vi "Get Cursor Position.vi"(8 "Logarithm?":bool, 9 "Inverted?":bool, 10 "Range":cluster{"Max":sgl, "Min":sgl}, 11 "Cursor Value In":sgl) -> (3 "Cursor Value Out":sgl)   [LabVIEW 2017, in "3D Plot.lvclass"]
uses:
  <vilib>/Math Plots/3D Math Plots/3D Plot/3D Plot/3D Plot.lvclass
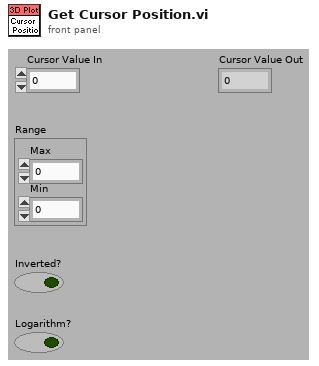
[diagram p1: front panel]
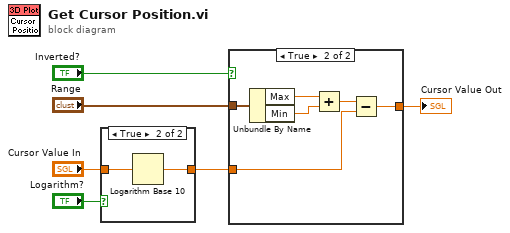
[diagram p0: block diagram]
diagram:
  n1 = case shown="True" "Logarithm?" {
    tunnel: "Cursor Value In" -> [w7 w9]
    tunnel: [w7 w8] -> w2
    frame False {
    }
    frame True {
      n2 = Logarithm Base 10(1:w9) -> (0:w8:sgl)
    }
  }
  n3 = case shown="True" "Inverted?" {
    tunnel: w2 -> [w10 w12]
    tunnel: [w10 w11] -> w1
    tunnel: "Range" -> [_ w16]
    frame False {
    }
    frame True {
      n4 = Unbundle By Name(w16) -> ("Max"=w15:sgl, "Min"=w14:sgl)
      n5 = Add(x=w15, y=w14) -> (x+y=w13:sgl)
      n6 = Subtract(x=w13, y=w12) -> (x-y=w11:sgl)
    }
  }
  "Cursor Value Out" <- w1
